vi "Obtain_Variable_Value.vi"(10 "JSON result":string="{\"result\":[[\"Position\",\"Speed\",\"Control\",\"error DAQ\",\"tiempo\",\"spPos\",\"spVel\",\"is late?\"],[9.99,0.000000,0.000000,\"Unsupported type of variable\",0.000000,0.000000,0.000000,false]]}") -> (3 "currentValue":dbl=9.99)   [LabVIEW 2015]
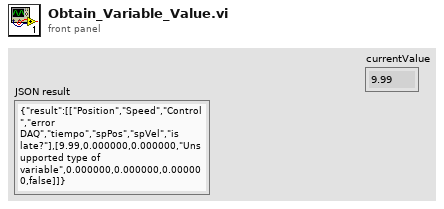
[diagram p1: front panel]
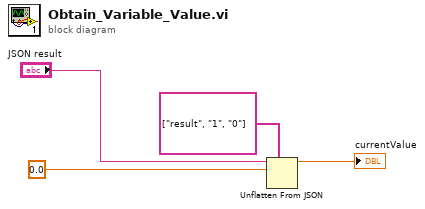
[diagram p0: block diagram]
diagram:
  n1 = Unflatten From JSON(path=string[] ["result", "1", "0"], JSON string="JSON result", type and defaults=0.0 ("Numeric")) -> (value=→"currentValue":dbl)  [unwired: 4 in, 1 out]
